vi "Sweep.vi"(6 "Last request":bool, 8 "error in (no error)":errorcluster, 11 "Spectrum Recorder in":refnum<class "Spectrum Recorder too.lvclass">) -> (0 "error out":errorcluster, 3 "Spectrum Recorder out":refnum<class "Spectrum Recorder too.lvclass">)   [LabVIEW 2018, in "Spectrum Recorder too.lvclass"]
uses:
  Spectrum Recorder too.lvclass
  C:/github/LabActor/Worker/Worker.lvclass
  Worker/Worker.lvclass/Worker.ctl
  Spectrum Recorder too.lvclass/Spectrum Recorder too.ctl
  Template Module/Read State.vi
  Read RP transceiver.vi
  Write RP transceiver.vi
  NHMFL_Core/Libraries/Red Pitaya/RP Core/RP Transceiver/RP Transceiver.lvclass
panel:
  out "Waveform Chart":dbl[](graph)
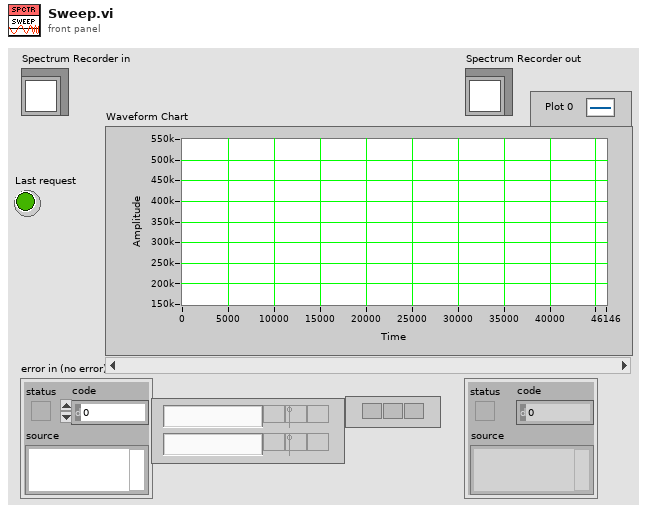
[diagram p1: front panel]
types:
  T1 = typedef "Worker State.ctl" = enum16{"Idle", "Starting", "Working", "Stopping"}
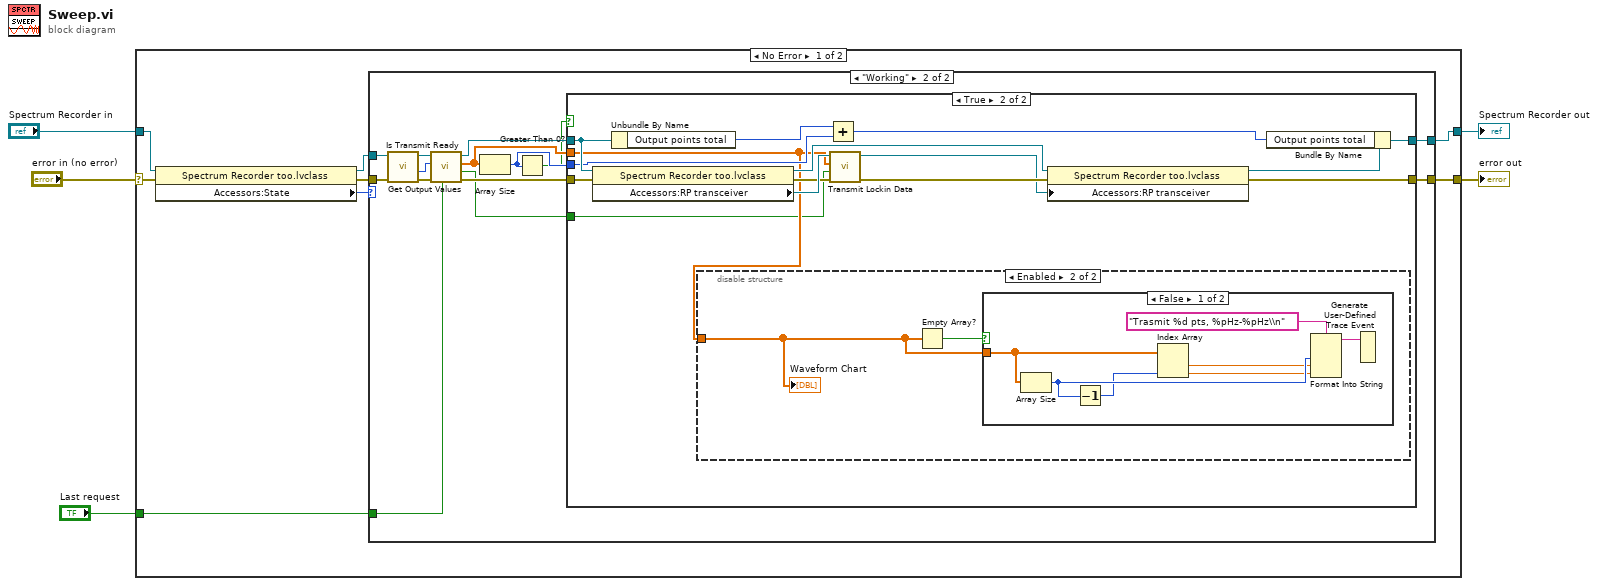
[diagram p0: block diagram]
diagram:
  n1 = case shown="No Error" "error in (no error)" {
    selector: "error in (no error)" -> [w12 w57]
    tunnel: [w11 w57] -> w4
    tunnel: [w13 w56] -> w2
    tunnel: "Spectrum Recorder in" -> [w9 w56]
    tunnel: "Last request" -> [w6 _]
    frame No Error {
      n2 = property class="Spectrum Recorder too.lvclass"(reference=w9, error in=w12) -> (reference out=w8:refnum<class "Spectrum Recorder too.lvclass">, error out=w10:errorcluster, "Accessors:State"=w7:T1)
      n3 = case shown="\"Working\"" w7 {
        tunnel: w8 -> [w15 w24]
        tunnel: w10 -> [w14 w22]
        tunnel: [w15 w28] -> w13
        tunnel: [w14 w27] -> w11
        tunnel: w6 -> [_ w26]
        frame "Idle", Default {
        }
        frame "Working" {
          n4 = call-dynamic "Is Transmit Ready.vi"("error in (no error)"=w22, "Spectrum Recorder too in"=w24) -> ("error out"=w21:errorcluster, "Unused buffer"=w17:i32, "Spectrum Recorder too out"=w23:refnum<class "Spectrum Recorder too.lvclass">)  [unwired: 6 in, 1 out]
          n5 = call-dynamic "Get Output Values.vi"("Last request"=w26, "error in (no error)"=w21, "Number of points"=w17, "Spectrum Recorder in"=w23) -> ("error out"=w20:errorcluster, "Reset"=w16:bool, "Output values"=w29:dbl[], "Spectrum Recorder out"=w19:refnum<class "Spectrum Recorder too.lvclass">)  [unwired: 4 in]
          n6 = Array Size(array=w29) -> (size(s)=w25:i32)
          n7 = Greater Than 0?(x=w25) -> (x > 0?=w18:bool)
          n8 = case shown="True" w18 {
            tunnel: w29 -> [_ w33]
            tunnel: [w31 w34] -> w28
            tunnel: [w30 w44] -> w27
            tunnel: w25 -> [_ w38]
            tunnel: w20 -> [w30 w42]
            tunnel: w19 -> [w31 w39]
            tunnel: w16 -> [_ w32]
            frame False {
            }
            frame True {
              n9 = property class="Spectrum Recorder too.lvclass"(reference=w39, error in=w42) -> (reference out=w36:refnum<class "Spectrum Recorder too.lvclass">, error out=w41:errorcluster, "Accessors:RP transceiver"=w46:refnum<class "RP Transceiver.lvclass">)
              n10 = Unbundle By Name(w39) -> ("Output points total"=w37:i64)
              n11 = disable-structure shown="Enabled" {
                disable-tunnel: w33 -> [_ w47]
                frame Disabled {
                }
                frame Enabled {
                  n12 = Empty Array?(array=w47) -> (empty?=w48:bool)
                  n13 = case shown="False" w48 {
                    tunnel: w47 -> [w54 _]
                    frame False {
                      n14 = Array Size(array=w54) -> (size(s)=w53:i32)
                      n15 = Decrement(x=w53) -> (x-1=w52:i32)
                      n16 = Index Array(array=w54, index #2=w52) -> (element #1=w51:dbl, element #2=w50:dbl)  [unwired: 1 in]
                      n17 = Format Into String(format string="Trasmit %d pts, %pHz-%pHz\\n", w53, w51, w50) -> (resulting string=w49:string)  [unwired: 2 in, 1 out]
                      n18 = Generate User-Defined Trace Event(2:w49) -> ()  [unwired: 1 in]
                    }
                    frame True {
                    }
                  }
                  "Waveform Chart" <- w47
                }
              }
              n19 = Add(x=w37, y=w38) -> (x+y=w40:i64)
              n20 = call-dynamic "Transmit Lockin Data.vi"("error in (no error)"=w41, "Reset"=w32, "Data"=w33, "RP Transceiver in"=w46) -> ("error out"=w45:errorcluster, "RP Transceiver out"=w43:refnum<class "RP Transceiver.lvclass">)  [unwired: 5 in, 1 out]
              n21 = property class="Spectrum Recorder too.lvclass"(reference=w36, error in=w45, "Accessors:RP transceiver"=w43) -> (reference out=w35:refnum<class "Spectrum Recorder too.lvclass">, error out=w44:errorcluster)
              n22 = Bundle By Name(cluster=w35, "Output points total"=w40) -> (w34:refnum<class "Spectrum Recorder too.lvclass">)
            }
          }
        }
      }
    }
    frame Error {
    }
  }
  "error out" <- w4
  "Spectrum Recorder out" <- w2
